vi "expose.vi"(8 "error in (no error)":errorcluster, 11 "Stresing_dual_cam in":refnum<class "Stresing_dual_cam.lvclass">) -> (0 "error out":errorcluster, 3 "Stresing_dual_cam out":refnum<class "Stresing_dual_cam.lvclass">)   [LabVIEW 2019, in "Stresing_dual_cam.lvclass"]
uses:
  Stresing_dual_cam.lvclass
  Stresing_dual_cam.lvclass/Stresing_dual_cam.ctl
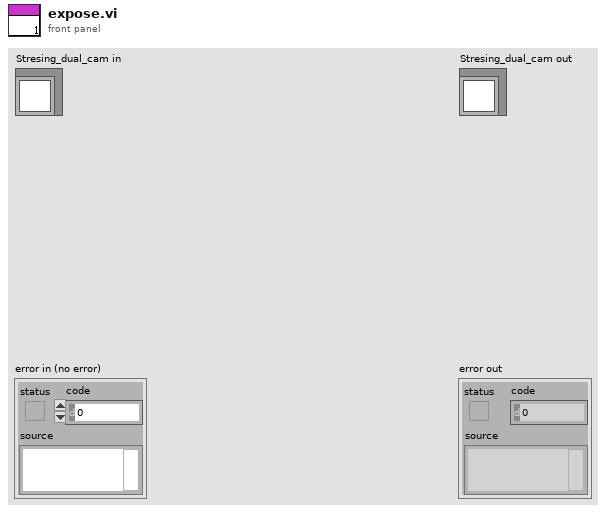
[diagram p1: front panel]
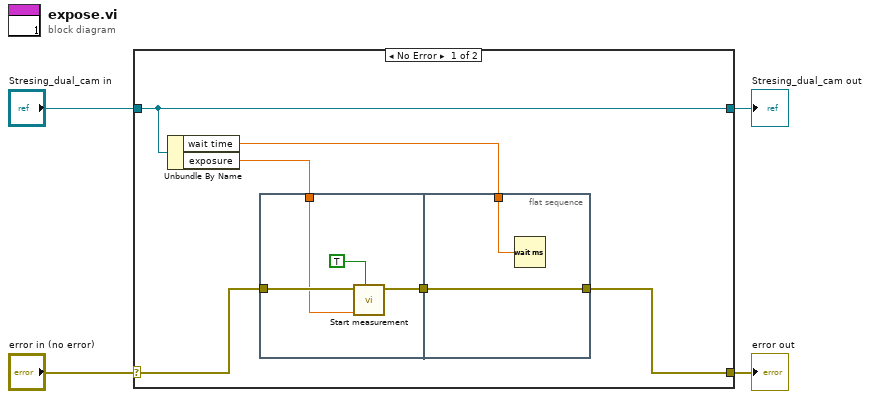
[diagram p0: block diagram]
diagram:
  n1 = case shown="No Error" "error in (no error)" {
    selector: "error in (no error)" -> [w10 w18]
    tunnel: [w9 w18] -> w3
    tunnel: [w7 w17] -> w1
    tunnel: "Stresing_dual_cam in" -> [w7 w17]
    frame No Error {
      n2 = Unbundle By Name(w7) -> ("wait time"=w6:dbl, "exposure"=w5:dbl)
      n3 = flat-sequence {
        tunnel: w10 -> [w14]
        tunnel: [w13] -> w8
        tunnel: w5 -> [w11]
        tunnel: [w16] -> w9
        tunnel: w8 -> [w16]
        tunnel: w6 -> [w15]
        frame #0 {
          n4 = call <instrlib>:"Start measurement.vi"("extTrig"=TRUE, "Exposure"=w11, "Camera error in"=w14) -> ("Camera error out"=w13:errorcluster)  [unwired: 6 in]
        }
        frame #1 {
          n5 = Wait (ms)(milliseconds to wait=w15) -> ()  [unwired: 1 out]
        }
      }
    }
    frame Error {
    }
  }
  "error out" <- w3
  "Stresing_dual_cam out" <- w1
